vi "Read connection.vi"(8 "error in (no error)":errorcluster, 11 "DbConnection in":refnum<class "ORM_DBC_dotNet.lvclass">) -> (0 "error out":errorcluster, 2 "connection":refnum<k24>, 3 "DbConnection out":refnum<class "ORM_DBC_dotNet.lvclass">)   [LabVIEW 2020, in "ORM_DBC_dotNet.lvlib" / "ORM_DBC_dotNet.lvclass"]
uses:
  ORM_DBC_dotNet.lvclass
  System.Data
  ORM_DBC_dotNet.lvclass/ORM_DBC_dotNet.ctl
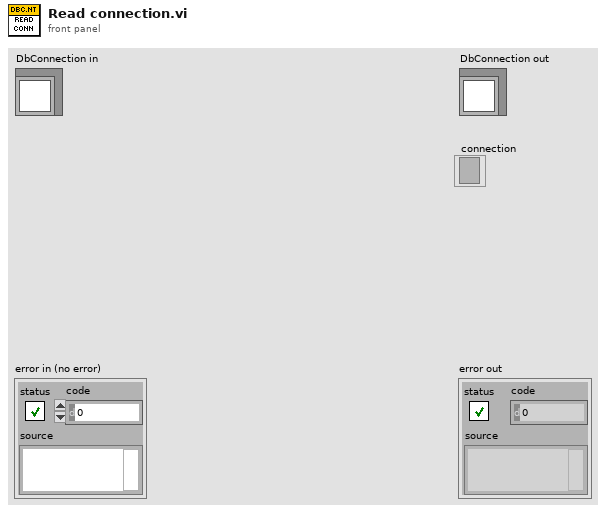
[diagram p1: front panel]
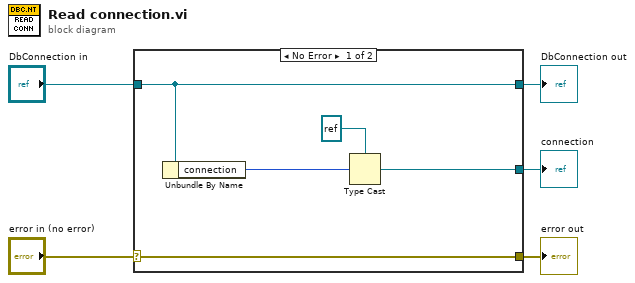
[diagram p0: block diagram]
diagram:
  n1 = case shown="No Error" "error in (no error)" {
    selector: "error in (no error)" -> [w10 w11]
    tunnel: [w10 w11] -> w4
    tunnel: [w9 w12] -> w2
    tunnel: "DbConnection in" -> [w9 w12]
    tunnel: [w7 _] -> w1
    frame No Error {
      n2 = Unbundle By Name(w9) -> ("connection"=w8:u64)
      n3 = Type Cast(type=refnum<k24> refnum ("connection"), x=w8) -> (*(type *) &x=w7:refnum<k24>)
    }
    frame Error {
    }
  }
  "error out" <- w4
  "DbConnection out" <- w2
  "connection" <- w1
